vi "Read Array (Voltage).vi"(0 "VISA resource name":refnum<visa-resource-name>, 11 "error in (no error)":errorcluster) -> (4 "VISA resource name out":refnum<visa-resource-name>, 6 "Samples (V)":dbl[](array[numeric]), 15 "error out":errorcluster)   [LabVIEW 2012, in "NH Research Regenerative Test Series.lvlib"]
doc: "Initiates a measurement and returns an array containing the instantaneous input voltage in Volts. Query Number of Samples is called internally after the measurement has been initiated to read how many samples are available to read from the instruments buffer.\n\nWaveforms are captured with every initiated measurement based on the Set Aperture Length.vi and Set Number of Samples.vi commands."
uses:
  <instrlib>/NH Research Regenerative Test Series/NH Research Regenerative Test Series.lvlib
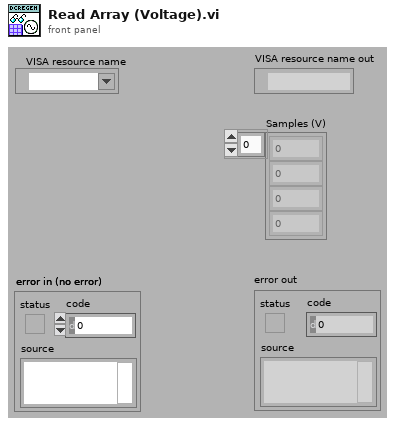
[diagram p1: front panel]
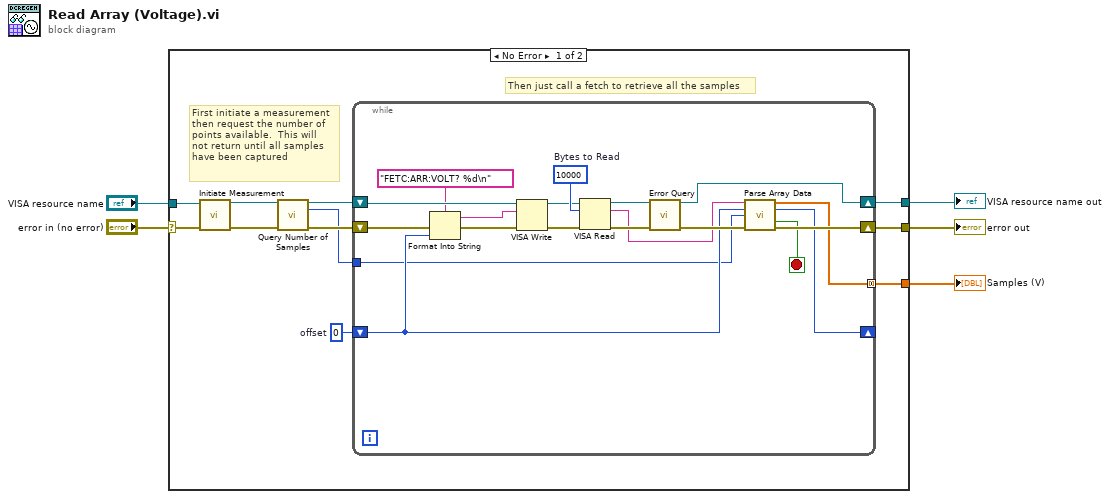
[diagram p0: block diagram]
diagram:
  n1 = case shown="No Error" "error in (no error)" {
    selector: "error in (no error)" -> [w12 w37]
    tunnel: [w15 w37] -> w4
    tunnel: [w16 w36] -> w1
    tunnel: "VISA resource name" -> [w11 w36]
    tunnel: [w14 _] -> w2
    frame No Error {
      w13 = 0  # offset
      # "Then just call a fetch to retrieve all the samples"
      # "First initiate a measurement\nthen request the number of\npoints available.  This will\nnot return until all samples\nhave been captured"
      n2 = call <instrlib>:"Initiate Measurement.vi"("VISA resource name"=w11, "error in (no error)"=w12) -> ("VISA resource name out"=w9:refnum<visa-resource-name>, "error out"=w10:errorcluster)  [unwired: 12 in]
      n3 = call <instrlib>:"Query Number of Samples.vi"("VISA resource name"=w9, "error in (no error)"=w10) -> ("VISA resource name out"=w8:refnum<visa-resource-name>, "Number of Samples"=w6:u32, "error out"=w7:errorcluster)  [unwired: 11 in]
      n4 = while {
        shift-right: [w24] -> w15
        shift-left: w7 -> [w28]
        shift-right: [w17] -> w16
        shift-left: w8 -> [w32]
        tunnel: [w19] -> w14 mode=concatenating
        shift-right: [w20] -> _
        shift-left: w13 -> [w22]
        tunnel: w6 -> [w21]
        stop <- w18 stop-if-true
        w35 = u32 10000  # Bytes to Read
        n5 = Format Into String(format string="FETC:ARR:VOLT? %d\n", error in=w28, w22) -> (resulting string=w26:string, error out=w27:errorcluster)  [unwired: 1 in]
        n6 = VISA Write(VISA resource name=w32, write buffer=w26, error in (no error)=w27) -> (VISA resource name out=w33:refnum<visa-resource-name>, error out=w34:errorcluster)  [unwired: 1 out]
        n7 = VISA Read(VISA resource name=w33, byte count=w35, error in (no error)=w34) -> (VISA resource name out=w31:refnum<visa-resource-name>, read buffer=w23:string, error out=w30:errorcluster)  [unwired: 1 out]
        n8 = call <instrlib>:"Error Query.vi"("VISA resource name"=w31, "error in (no error)"=w30) -> ("VISA resource name out"=w17:refnum<visa-resource-name>, "error out"=w25:errorcluster)  [unwired: 10 in, 2 out]
        n9 = call <instrlib>:"Parse Array Data.vi"("Samples String"=w23, "Current Index"=w22, "Number of Samples"=w21, "error in (no error)"=w25) -> ("Samples"=w19:dbl[], "Next Index"=w20:i32, "Stop Reading Samples"=w18:bool, "error out"=w24:errorcluster)  [unwired: 8 in]
      }
    }
    frame Error {
    }
  }
  "error out" <- w4
  "VISA resource name out" <- w1
  "Samples (V)" <- w2
